vi "Define Target.vi"(8 "error in (no error)":errorcluster, 10 "Core":refnum<class "Sequencer Core.lvclass">, 11 "Instrument Sequencer Sender in":refnum<class "Instrument Sequencer Sender Msg.lvclass">) -> (0 "error out":errorcluster, 3 "Instrument Sequencer Sender out":refnum<class "Instrument Sequencer Sender Msg.lvclass">)   [LabVIEW 2020, in "Instrument Handler.lvlib" / "Instrument Sequencer Sender Msg.lvclass"]
doc: "Populate the Instrument Sequencer Sender Msg."
uses:
  Instrument Sequencer Sender Msg.lvclass
  PPL/HDH.Actor Framework.Core.Sequencer.lvlibp/Sequencer Core/Sequencer Core.lvclass
  Instrument Sequencer Sender Msg.lvclass/Instrument Sequencer Sender Msg.ctl
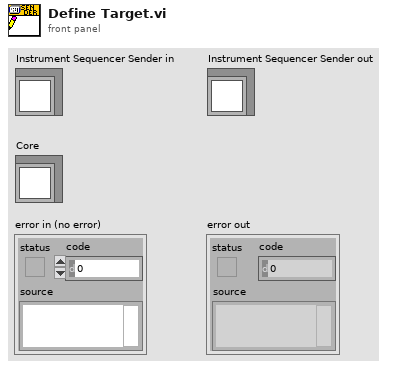
[diagram p1: front panel]
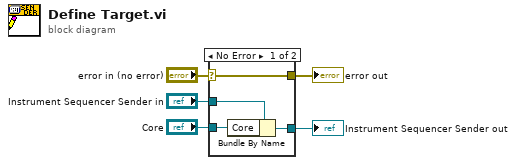
[diagram p0: block diagram]
diagram:
  n1 = case shown="No Error" "error in (no error)" {
    selector: "error in (no error)" -> [w9 w10]
    tunnel: [w9 w10] -> w4
    tunnel: [w7 w11] -> w2
    tunnel: "Instrument Sequencer Sender in" -> [w8 w11]
    tunnel: "Core" -> [w6 _]
    frame No Error {
      n2 = Bundle By Name(cluster=w8, "Core"=w6) -> (w7:refnum<class "Instrument Sequencer Sender Msg.lvclass">)
    }
    frame Error {
    }
  }
  "error out" <- w4
  "Instrument Sequencer Sender out" <- w2
